vi "Upload Package to SystemLink Repository (Async).vi"(0 "SystemLink repo in":T1, 5 "package filepath":path, 9 "timeout (ms) (10000)":u32=10000, 11 "error in (no error)":errorcluster) -> (4 "SystemLink repo out":T1, 6 "jobID":string, 15 "error out":errorcluster)   [LabVIEW 2017, in "SystemLink_Repo_API.lvlib"]
doc: "Uploads the package to the SystemLink repository. This VI sends this command asynchronously, which means this VI sends this command and returns without waiting for the command to finish executing on the SystemLink server.\n\nInputs:\nPackage filepath - This is the filepath of the package (.nipkg, .ipk) you want to upload.\n\nOutputs:\njobID - Returns the job ID that corresponds to this upload command.\n\nError Handling:\nOutputs Error 6000 if the upload job fails.\nOutputs Error 6001 if the upload job does not return a status of \"succeeded\" or \"failed\" within the timeout period."
uses:
  SystemLink_Repo_API.lvlib
  systemlink repo.ctl
  <vilib>/httpClient/ClientHandle.ctl
  <vilib>/httpClient/MultipartData.ctl
  063236bb-0006-43ce-b9fa-a45e1a69d032.vi
  <vilib>/JDP Science/JSONtext/Find Item.vi
  <vilib>/JDP Science/JSONtext/String Subset.vi
  <vilib>/JDP Science/JSONtext/Parsing/Parse Full Path or Item Name.vi
  <vilib>/JDP Science/JSONtext/Offset/Find Item Locations by Path.vi
  <vilib>/JDP Science/JSONtext/JSON text to Variant.vi
  <vilib>/httpClient/LabVIEWHTTPClient.lvlib
panel:
  out "body":string
  out "headers":string
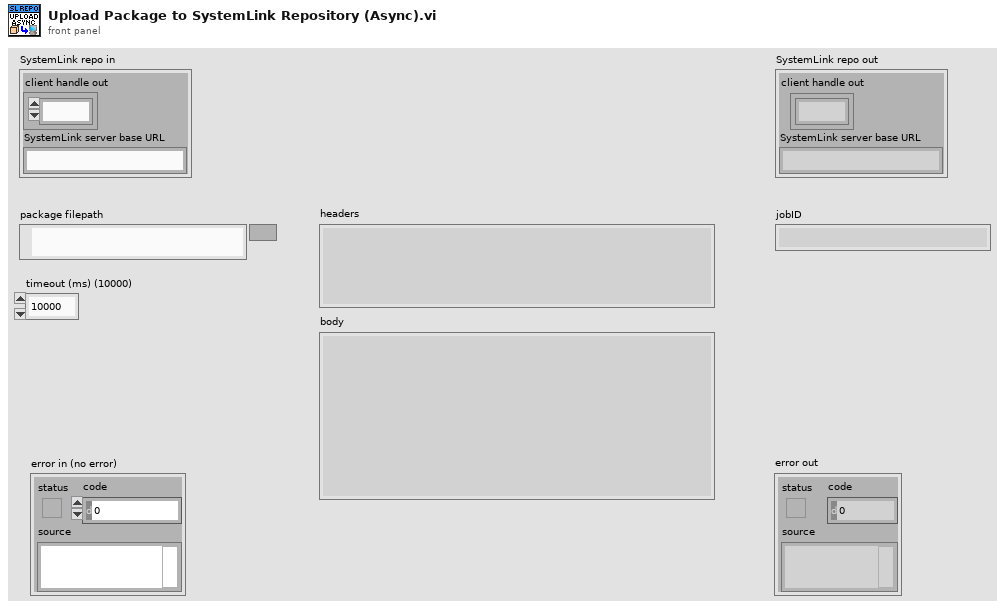
[diagram p1: front panel]
types:
  T1 = typedef "SystemLink_Repo_API.lvlib/systemlink repo.ctl" = cluster{"client handle out":T2, "SystemLink server base URL":string}
  T2 = typedef "LabVIEWHTTPClient.lvlib/ClientHandle.ctl" = refnum<k1>
  T3 = typedef "LabVIEWHTTPClient.lvlib/MultipartData.ctl" = cluster{"Name":string, "Value":string, "File":path, "Filename":string, "MIME type":string}
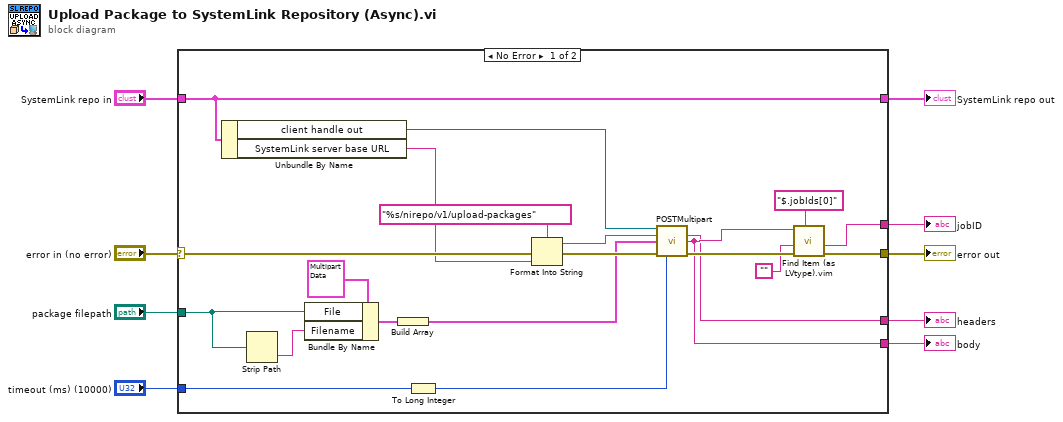
[diagram p0: block diagram]
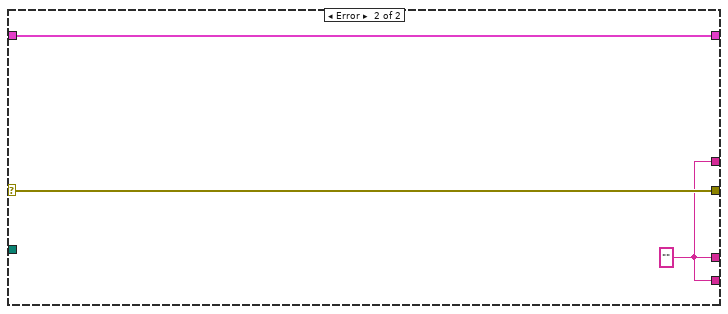
[diagram p2: hidden frame]
diagram:
  n1 = case shown="No Error" "error in (no error)" {
    selector: "error in (no error)" -> [w27 w33]
    tunnel: "SystemLink repo in" -> [w12 w31]
    tunnel: [w24 w33] -> w8
    tunnel: [w14 w32] -> w4
    tunnel: [w20 w32] -> w7
    tunnel: [w19 w32] -> w6
    tunnel: "package filepath" -> [w13 _]
    tunnel: [w12 w31] -> w2
    tunnel: "timeout (ms) (10000)" -> [w11 _]
    frame No Error {
      n2 = Unbundle By Name(w12) -> ("client handle out"=w28:T2, "SystemLink server base URL"=w21:string)
      n3 = Strip Path(path=w13) -> (name=w16:string)  [unwired: 1 out]
      n4 = Bundle By Name(cluster=T3 {"Name"="test package", "Value"="", "File"=path "", "Filename"="", "MIME type"="application/octet-stream"} ("Element"), "File"=w13, "Filename"=w16) -> (w17:T3)
      n5 = Build Array(w17) -> (w15:T3[])
      n6 = To Long Integer(number=w11) -> (32bit integer=w10:i32)
      n7 = Format Into String(format string="%s/nirepo/v1/upload-packages", error in=w27, w21) -> (resulting string=w29:string, error out=w26:errorcluster)  [unwired: 1 in]
      n8 = call <vilib>:"POSTMultipart.vi"("client handle"=w28, "url"=w29, "data"=w15, "error in (no error)"=w26, "timeout (10000)"=w10) -> ("headers"=w19:string, "body"=w20:string, "error out"=w25:errorcluster)  [unwired: 7 in, 1 out]
      n9 = call "Find Item (as LVtype).vim"("$Path or Item Name"="$.jobIds[0]", "error in (no error)"=w25, "Data Type and Default Value"="", "JSON"=w20) -> ("error out"=w24:errorcluster, "Data"=w14:string)  [unwired: 4 in, 2 out]
    }
    frame Error {
      w32 = "" ("headers")
    }
  }
  "error out" <- w8
  "SystemLink repo out" <- w2
  "headers" <- w6
  "body" <- w7
  "jobID" <- w4
